vi "Main Vending Machine.vi"() -> ()   [LabVIEW 2017]
uses:
  Controls/Pick up.ctl
  Controls/Refrescos.ctl
  Controls/Coins.ctl
panel:
  in  "Coins":T1
  in  "Items":T2
  in  "Change":bool
  out "Status":string
  out "Pick up":T3
  in  "stop":bool
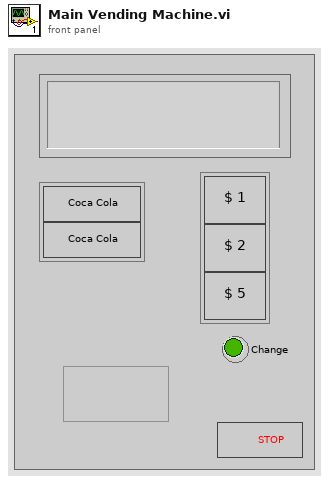
[diagram p1: front panel]
types:
  T1 = typedef "Coins.ctl" = cluster{"1 coin":bool, "2 coins":bool, "5 coins":bool}
  T2 = typedef "Refrescos.ctl" = cluster{"Option 1":bool, "Option 2":bool}
  T3 = typedef "Pick up.ctl" = bool
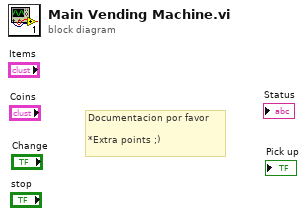
[diagram p0: block diagram]
diagram:
  # "Documentacion por favor\n\n*Extra points ;)"
